vi "FTW-SQLite-Transaction-End.vi"(0 "SQLite Connector":refnum<class "FTW-SQLite-Connector.lvclass">, 11 "error in":errorcluster) -> (4 "SQLite Connector out":refnum<class "FTW-SQLite-Connector.lvclass">, 6 "Time to Execute+Compile":dbl format="%.6fsec", 8 "Time to Compile SQL":dbl format="%.6fsec", 15 "error out":errorcluster)   [LabVIEW 2013, in "FTW-SQLite-Connector.lvclass"]
uses:
  FTW-SQLite-Connector.lvclass
panel:
  # "Inputs"
  # "Outputs"
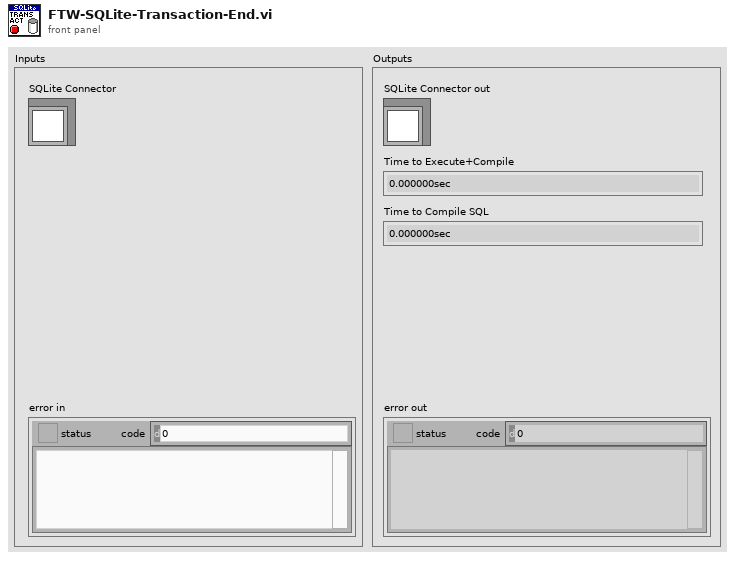
[diagram p1: front panel]
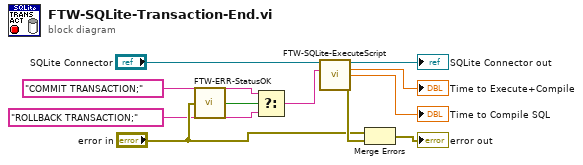
[diagram p0: block diagram]
diagram:
  n1 = call "FTW-ERR-StatusOK.vi"("error to check"="error in") -> ("Status OK?"=w4:bool)
  n2 = Select(t="COMMIT TRANSACTION;" ("SQL Script"), s=w4, f="ROLLBACK TRANSACTION;" ("SQL Script")) -> (s? t:f=w1:string)
  n3 = call "FTW-SQLite-ExecuteScript.vi"("SQLite Connector"="SQLite Connector", "SQL Script"=w1) -> ("SQLite Connector out"=→"SQLite Connector out":refnum<class "FTW-SQLite-Connector.lvclass">, "Time to Execute+Compile"=→"Time to Execute+Compile":dbl, "Time to Compile SQL"=→"Time to Compile SQL":dbl, "error out"=w11:errorcluster)  [unwired: 10 in]
  n4 = Merge Errors("error in", w11) -> (→"error out":errorcluster)
